vi "CMD_Harvester.vi"(1 "Line":string) -> (0 "Done":bool)   [LabVIEW 2015]
panel:
  in  "Parameters":i32[](array[numeric])=[1, 1, 1, 0, 0]
  in  "Subcommands":string[](array[string])=["at", "for", "until", "up", "down"]
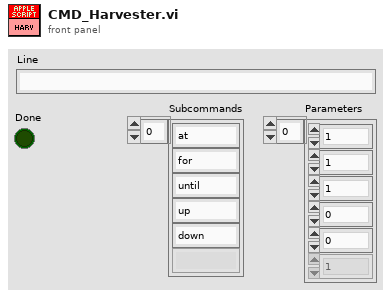
[diagram p1: front panel]
types:
  T1 = typedef "WPI_MotorControlDeviceRef.ctl" = cluster{"DeviceStatus":errorcluster, "Type":T2, "PWM":cluster{"PWM Channel":T3, "DeadBand":T4}, "CAN":cluster{"Device Number":u8, "Control Mode":T5, "Semaphore":T6, "Max Vout":dbl, "TalonSRX Control Mode":T7}, "Invert":bool}
  T2 = typedef "WPI_MotorControlType.ctl" = enum16{"PWM", "CAN", "CANTalonSRX"}
  T3 = typedef "FPGA_DIOPWMChannel.ctl" = enum8{"PWM 0", "PWM 1", "PWM 2", "PWM 3", "PWM 4", "PWM 5", "PWM 6", "PWM 7", "PWM 8", "PWM 9", "PWM MXP 0", "PWM MXP 1", "PWM MXP 2", "PWM MXP 3", "PWM MXP 4", "PWM MXP 5", "PWM MXP 6", "PWM MXP 7", "PWM MXP 8", "PWM MXP 9", "Invalid"}
  T4 = typedef "WPI_PWMDeadband.ctl" = cluster{"Name":string, "maxPositivePwm":i32, "minPositivePwm":i32, "centerPwm":i32, "maxNegativePwm":i32, "minNegativePwm":i32, "angularRange":u16}
  T5 = typedef "WPI_CANJaguar_ControlMode.ctl" = enum8{"Percent VBus", "Current", "Speed", "Position", "Voltage"}
  T6 = typedef "Semaphore RefNum" = refnum<k1>
  T7 = typedef "WPI_CANTalonSRX_APIControlMode.ctl" = enum8{"Percent VBus", "Speed", "Position", "Slave", "Unchanged / Invalid", "Voltage Compensation", "Current", "Motion Profile"}
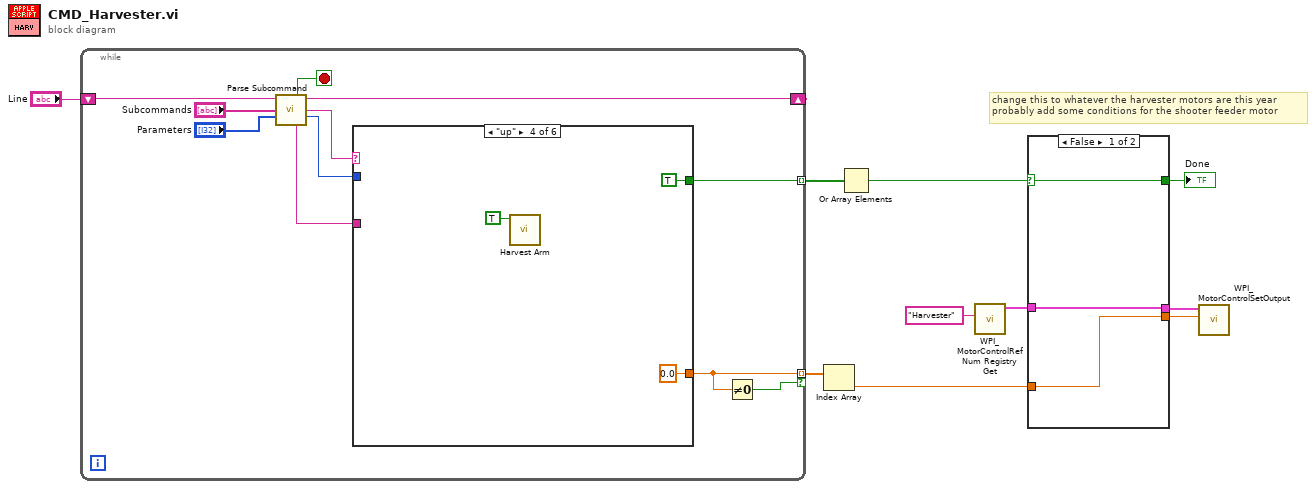
[diagram p0: block diagram]
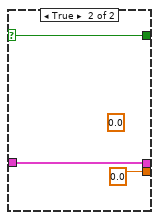
[diagram p2: hidden frame]
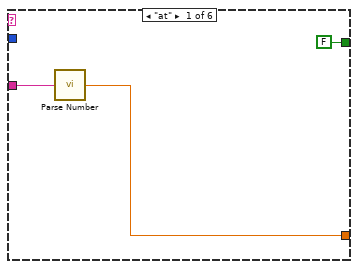
[diagram p3: hidden frame]
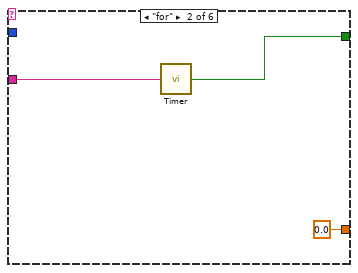
[diagram p4: hidden frame]
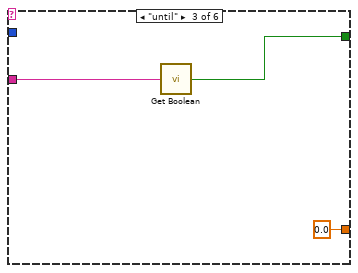
[diagram p5: hidden frame]
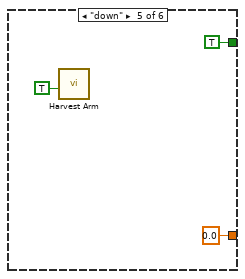
[diagram p6: hidden frame]
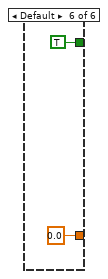
[diagram p7: hidden frame]
diagram:
  # "change this to whatever the harvester motors are this year\nprobably add some conditions for the shooter feeder motor"
  n1 = while {
    shift-right: [w18] -> _
    shift-left: "Line" -> [w21]
    tunnel: [w13] -> w9 mode=indexing
    tunnel: [w12] -> w8 mode=indexing if=w11
    stop <- w17 stop-if-true
    n2 = call "Parse Subcommand.vi"("Text In"=w21, "Subcommands"="Subcommands", "Parameters"="Parameters") -> ("Done"=w17:bool, "Text Out"=w18:string, "Subcommand"=w16:string, "# of Parameters"=w15:i32, "Parameter 1"=w14:string)  [unwired: 6 in, 2 out]
    n3 = case shown="\"up\"" w16 {
      tunnel: w15 -> [_ _ _ _ _ _]
      tunnel: w14 -> [w24 w27 w30 _ _ _]
      tunnel: [FALSE ("Value") w25 w28 TRUE ("Value") TRUE ("Value") TRUE ("Value")] -> w13
      tunnel: [w22 0.0 ("Number") 0.0 ("Number") 0.0 ("Number") 0.0 ("Number") 0.0 ("Number")] -> w12
      frame "at" {
        n4 = call "Parse Number.vi"("String"=w24) -> ("Number"=w22:dbl)
      }
      frame "for" {
        n5 = call "Timer.vi"("Seconds (string)"=w27) -> ("Done"=w25:bool)
      }
      frame "until" {
        n6 = call "Get Boolean.vi"("Name"=w30) -> ("Value"=w28:bool)
      }
      frame "up" {
        n7 = call "Harvest Arm.vi"("Arm Up"=TRUE) -> ()  [unwired: 11 in]
      }
      frame "down" {
        n8 = call "Harvest Arm.vi"("Arm Down"=TRUE) -> ()  [unwired: 11 in]
      }
      frame Default {
      }
    }
    n9 = Not Equal To 0?(x=w12) -> (x != 0?=w11:bool)
  }
  n10 = Index Array(array=w8) -> (element=w3:dbl)  [unwired: 1 in]
  n11 = Or Array Elements(Boolean array=w9) -> (logical OR=w7:bool)
  n12 = call <vilib>:"WPI_MotorControlRefNum Registry Get.vi"("refnum name"="Harvester") -> ("MotorControlDevRef"=w5:T1)  [unwired: 9 in, 1 out]
  n13 = case shown="False" w7 {
    selector: w7 -> [w41 w44]
    tunnel: [w41 w44] -> w6
    tunnel: w5 -> [w40 w43]
    tunnel: [w40 w43] -> w4
    tunnel: w3 -> [w39 _]
    tunnel: [w39 0.0] -> w2
    frame False {
    }
    frame True {
      (unwired) 0.0
    }
  }
  "Done" <- w6
  n14 = call <vilib>:"WPI_MotorControlSetOutput.vi"("Output"=w2, "MotorControlDevRef"=w4) -> ()  [unwired: 7 in, 3 out]
